vi "CCD photon image_Shaowei.vi"() -> ()   [LabVIEW 2009]
uses:
  <vilib>/Utility/file.llb/Read From Spreadsheet File (DBL).vi
  Instance           5 35Saved   CCD photon image_540_800_CR .vi
  Instance           4 35Saved   CCD photon image_540_800_CR .vi
  Instance           3 35Saved   CCD photon image_540_800_CR .vi
  Instance           8 35Saved   CCD photon image_540_800_CR .vi
  <vilib>/Analysis/Matrix/Numeric/Conversions/Array To Matrix - RA2.vi
  Instance          12 35Saved   CCD photon image_540_800_CR .vi
  Instance          15 35Saved   CCD photon image_540_800_CR .vi
  Instance          18 35Saved   CCD photon image_540_800_CR .vi
  Instance          21 35Saved   CCD photon image_540_800_CR .vi
  Instance          25 35Saved   CCD photon image_540_800_CR .vi
  Instance          24 35Saved   CCD photon image_540_800_CR .vi
  <vilib>/Analysis/Matrix/NI_Matrix.lvlib
panel:
  in  "?":bool
  in  "?":path=path "C:/Users/S. W. Li/Desktop/0463-730.lvm"
  in  "?":path=path "D:/Untitled.txt"
  in  "?":path
  in  "stop 2":bool
  in  "#6":bool
  in  "#5":bool
  in  "?":bool
  in  "stop":bool
  in  "?":ext=1340.0
  in  "to":dbl=950.0
  in  "From":dbl=550.0
  out "Intensity Graph 6":dbl[][](graph)
  out "Col":dbl
  out "to":dbl
  out "Matrix 6":string
  in  "lstart (nm)":dbl
  in  "lend (nm)":dbl
  out "eV":dbl
  out "eV":dbl
  out "Intensity Graph 5":dbl[][](graph)
  out "Col":dbl
  out "to":dbl
  out "Matrix 5":string
  in  "lstart (nm)":dbl
  in  "lend (nm)":dbl
  out "eV":dbl
  out "eV":dbl
  in  "?":bool
  out "MAX":dbl
  out "MIN":dbl
  out "X":sgl
  out "Y":sgl
  out "to":dbl
  out "Col":dbl
  out "eV":dbl
  out "eV":dbl
  in  "lend (nm)":dbl
  in  "lstart (nm)":dbl
  out "eV":dbl
  out "eV":dbl
  in  "lend (nm)":dbl
  in  "lstart (nm)":dbl
  out "to":dbl
  out "Col":dbl
  out "to":dbl
  out "Col":dbl
  out "eV":dbl
  out "eV":dbl
  in  "lend (nm)":dbl
  in  "lstart (nm)":dbl
  in  "?":dbl=32.0
  out "eV":dbl
  out "eV":dbl
  in  "lend (nm)":dbl
  in  "lstart (nm)":dbl
  out "to":dbl
  out "Col":dbl
  in  "#3":bool
  in  "#4":bool
  in  "#2":bool
  out "Intensity Graph 4":dbl[][](graph)
  out "Matrix 4":string
  out "Intensity Graph 3":dbl[][](graph)
  out "Matrix 3":string
  out "Matrix 2":string
  out "Intensity Graph 2":dbl[][](graph)
  out "Matrix 1":string
  out "Intensity Graph":dbl[][](graph)
  # "Input File"
  # "2 Files"
  # "1 File"
  # "1st"
  # "2nd"
  # "Spectra Range"
  # "nm"
  # "nm"
  # "# of Pixel"
  # "Image Size"
  # "Bit"
  # "Active Matrix"
  # "ON"
  # "OFF"
  # "Cosmic Ray Removal"
  # "NO"
  # "YES"
  # "Value"
  # "Position"
  # "Save File"
  # "NO"
  # "YES"
  # "File Name"
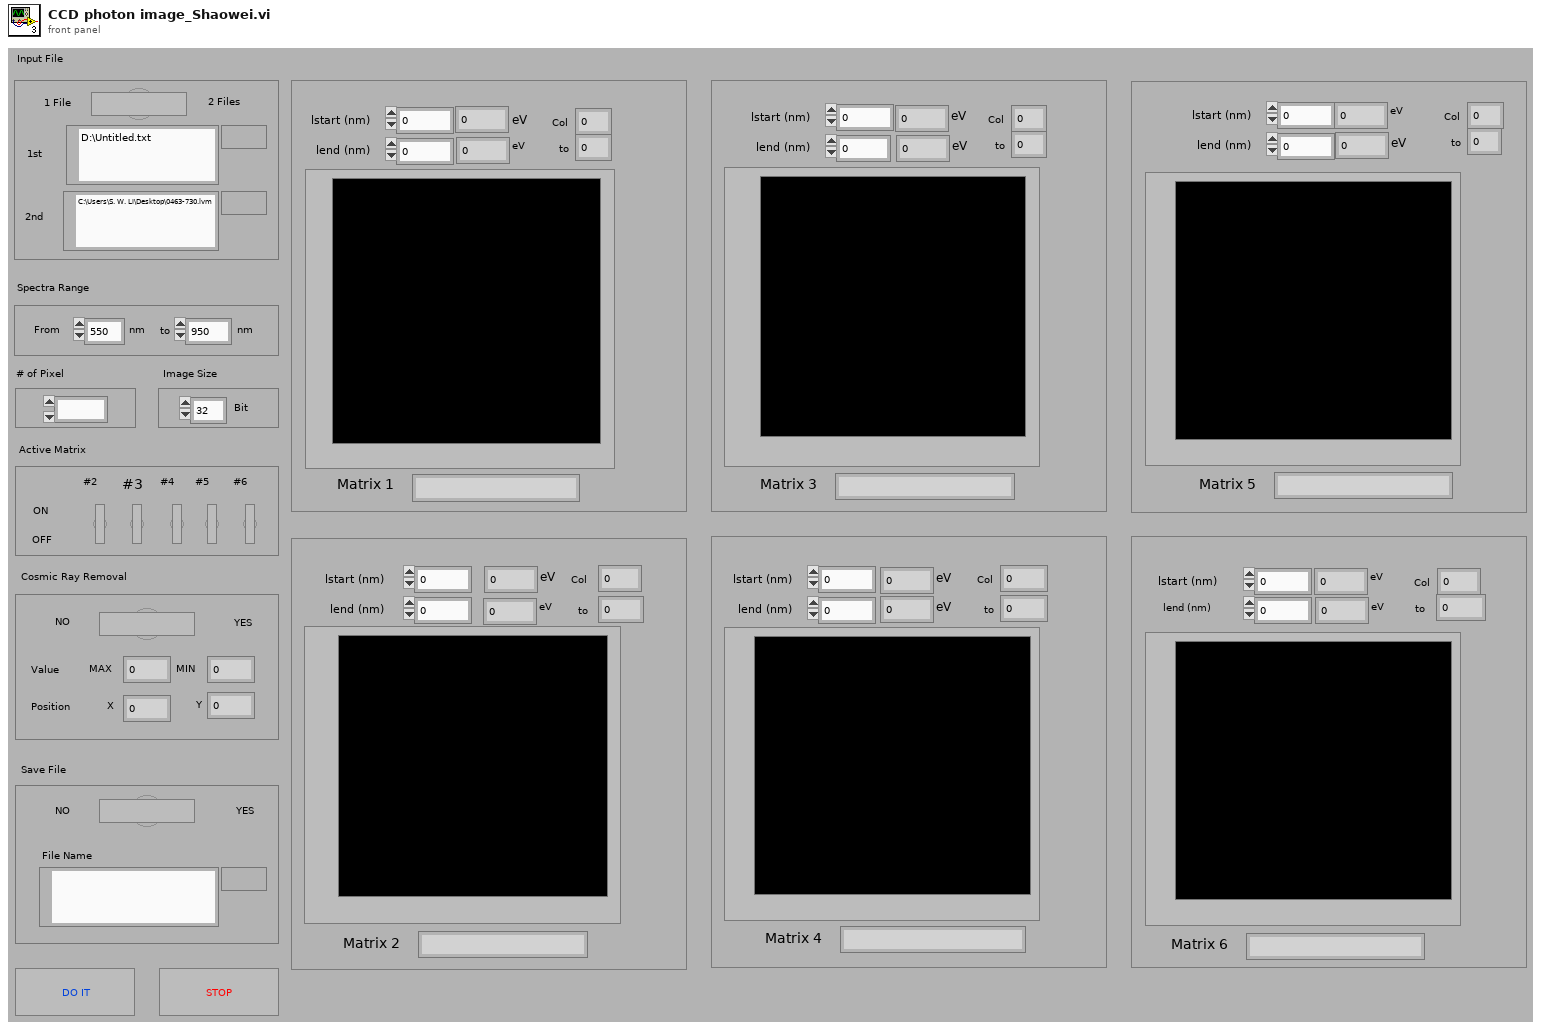
[diagram p1: front panel]
types:
  T1 = typedef "NI_Matrix.lvlib/RealMatrix.ctl" = dbl[][]
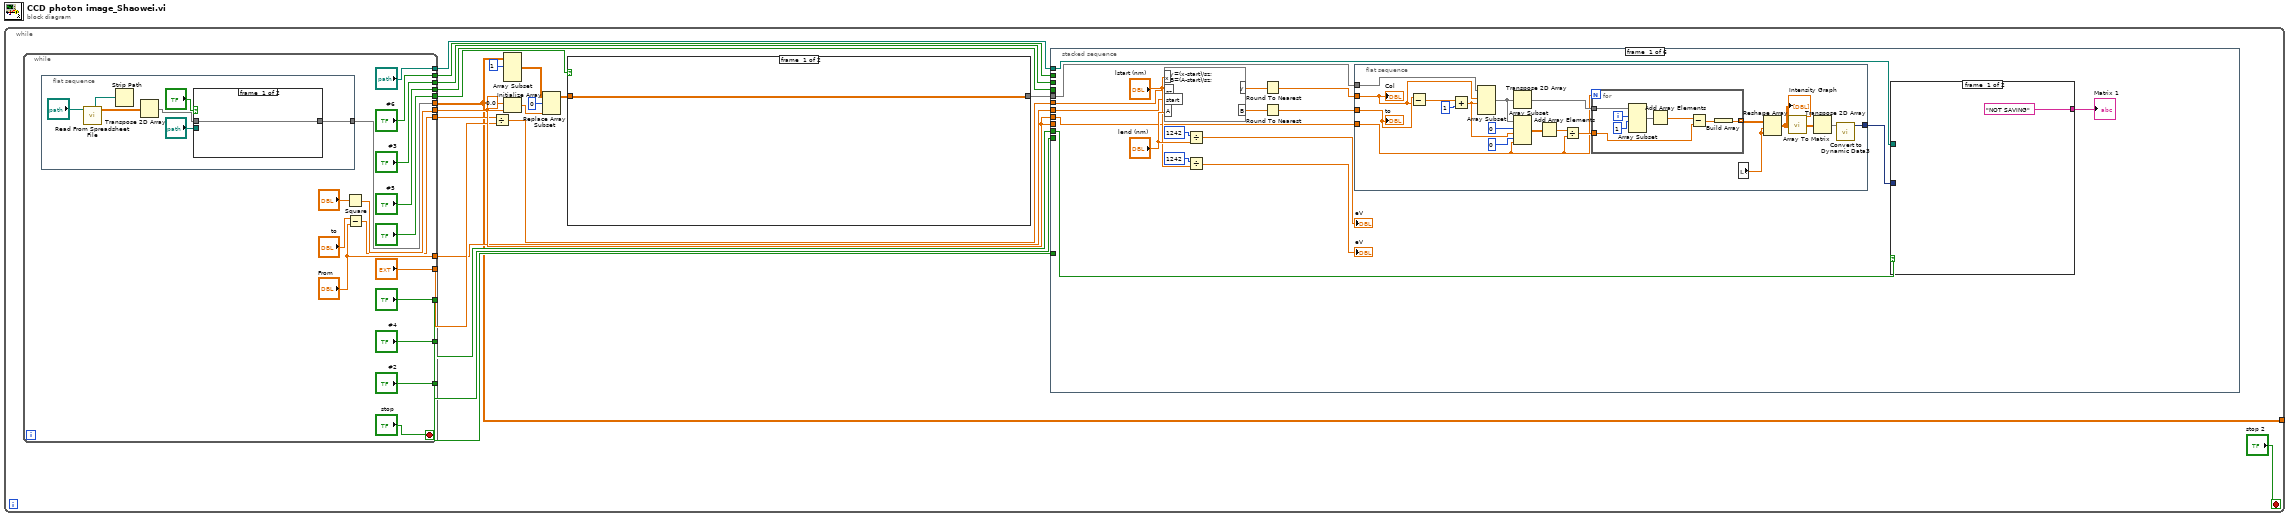
[diagram p0: block diagram]
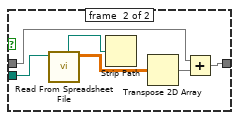
[diagram p2: hidden frame]
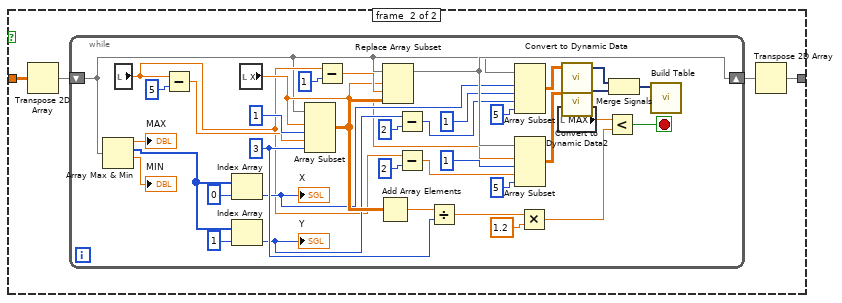
[diagram p3: hidden frame]
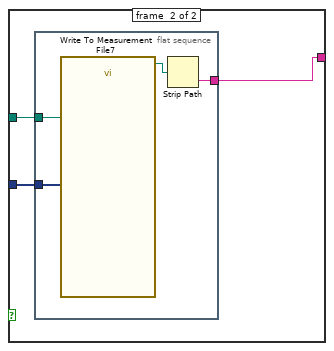
[diagram p4: hidden frame]
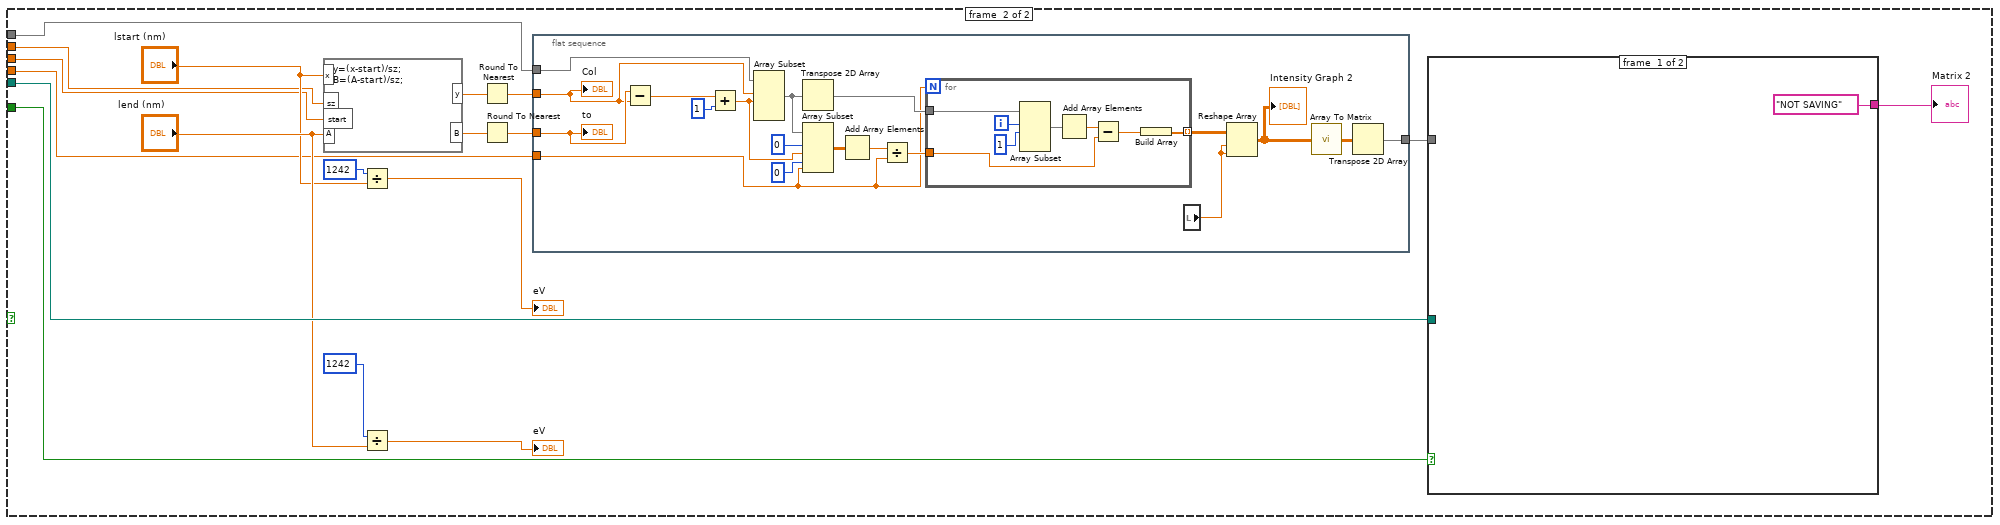
[diagram p6: hidden frame]
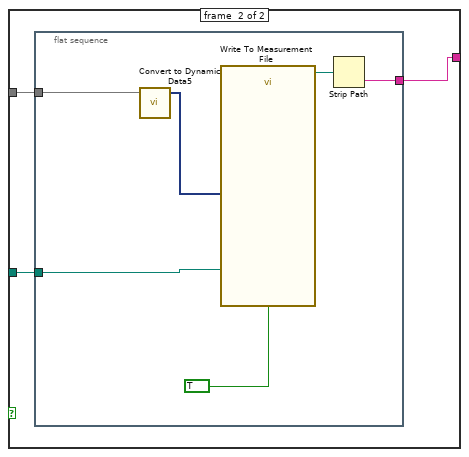
[diagram p7: hidden frame]
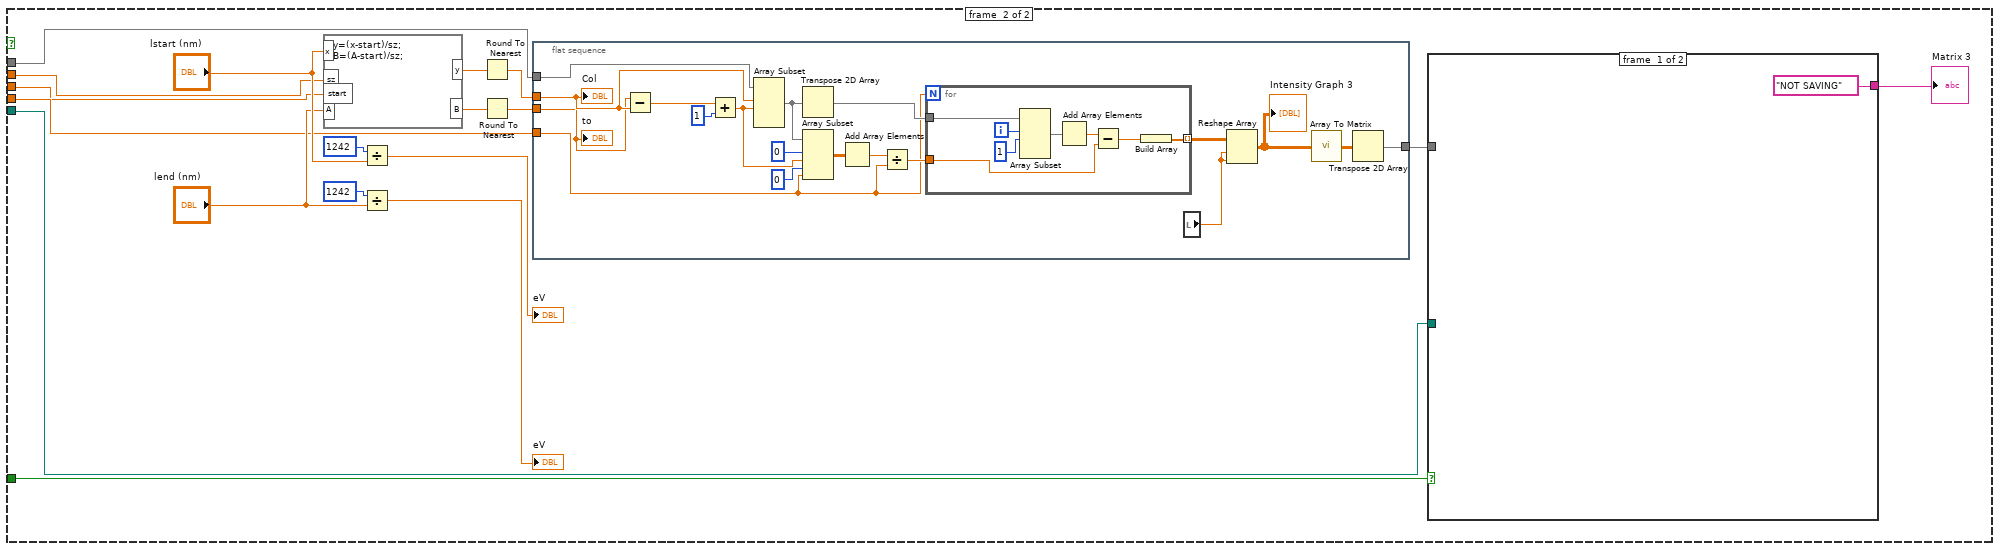
[diagram p9: hidden frame]
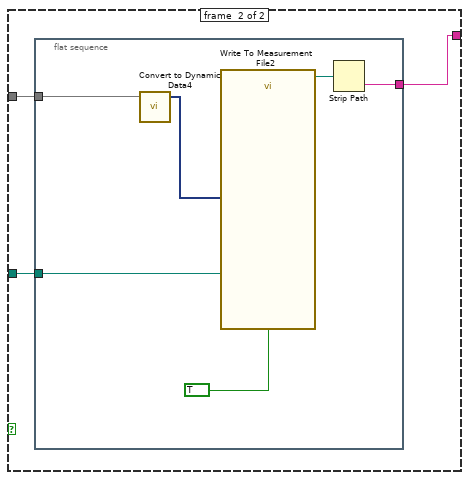
[diagram p10: hidden frame]
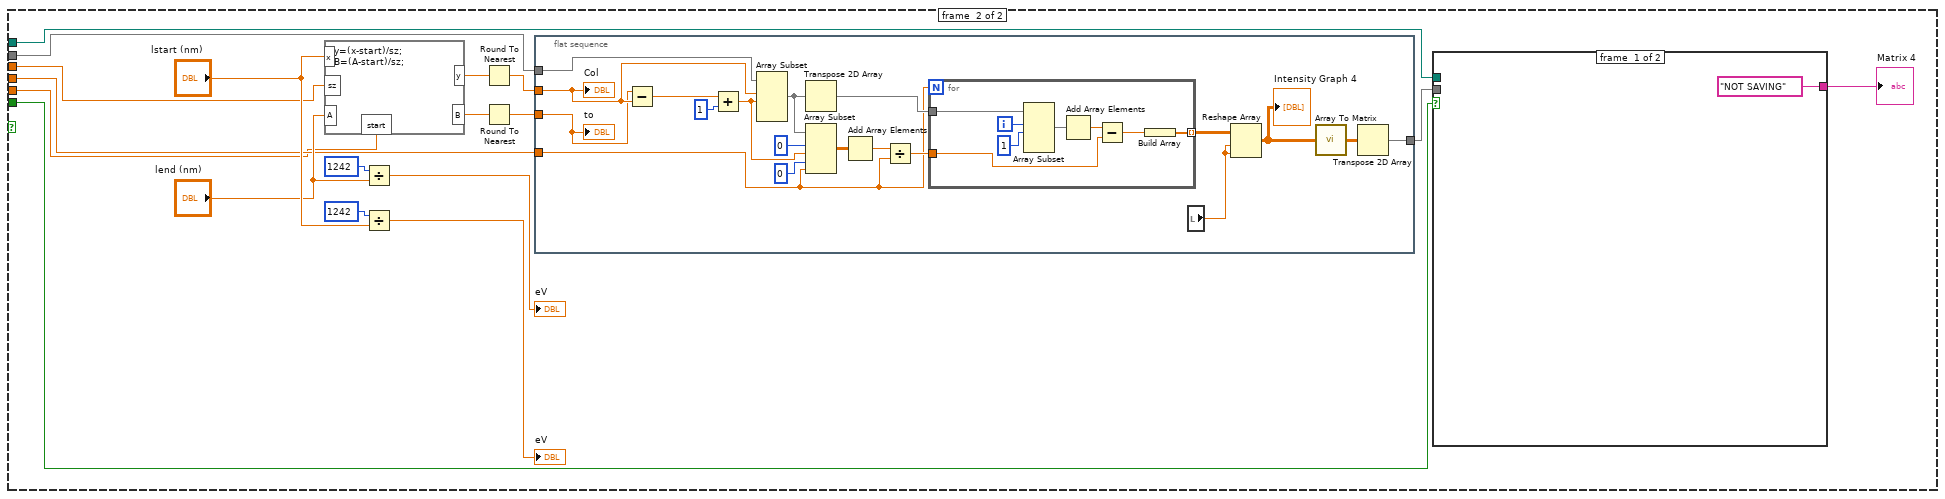
[diagram p12: hidden frame]
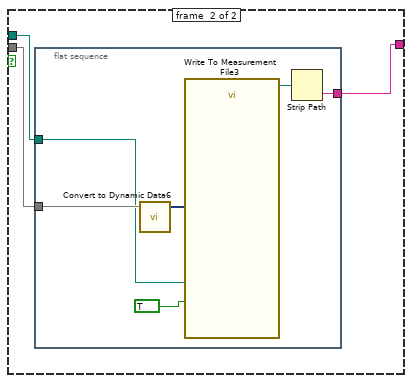
[diagram p13: hidden frame]
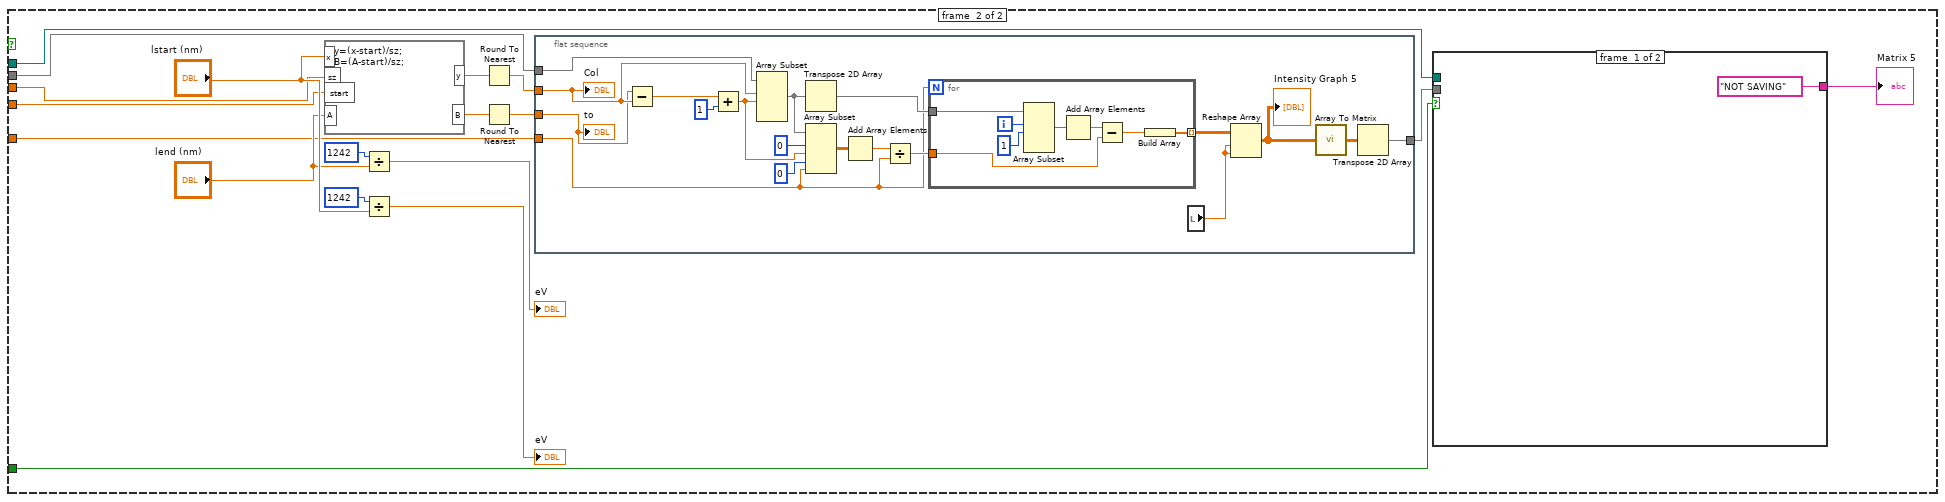
[diagram p15: hidden frame]
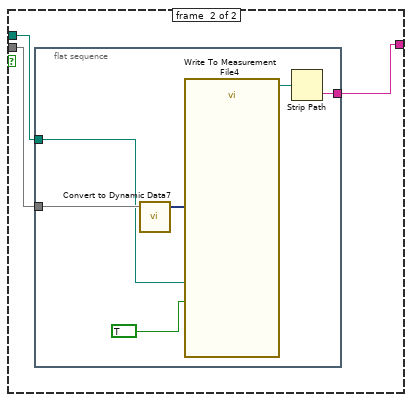
[diagram p16: hidden frame]
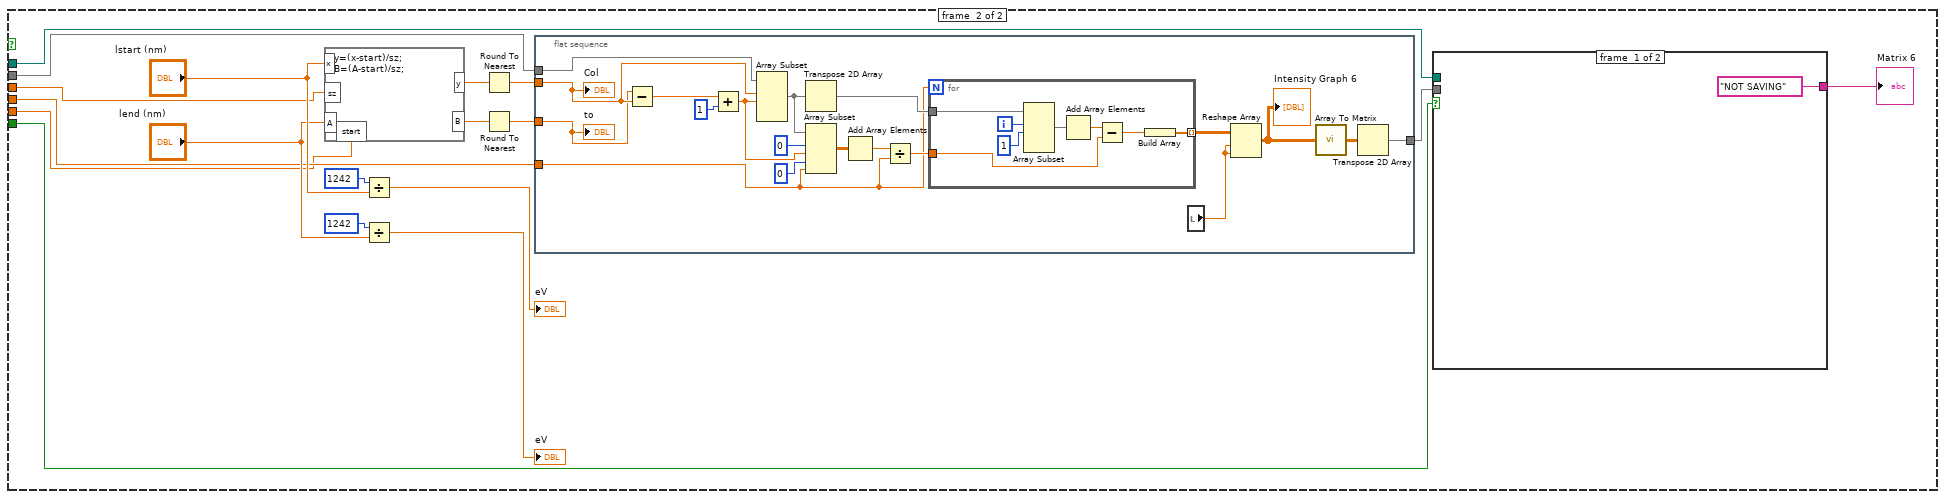
[diagram p18: hidden frame]
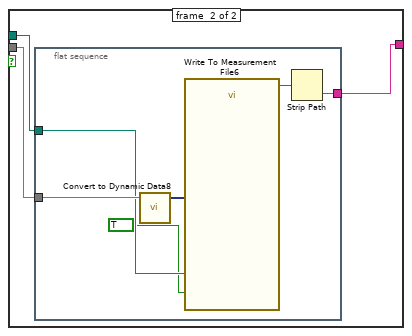
[diagram p19: hidden frame]
diagram:
  n1 = while {
    tunnel: [w2] -> _
    stop <- "stop 2" stop-if-true
    n2 = while {
      tunnel: ["?"] -> w1
      tunnel: ["#4"] -> w22
      tunnel: ["#3"] -> w21
      tunnel: ["#2"] -> w20
      tunnel: [w34] -> w14
      tunnel: ["?"] -> w11
      tunnel: ["?"] -> w10
      tunnel: [w30] -> w9
      tunnel: ["From"] -> w3
      tunnel: ["?"] -> w7
      tunnel: ["#5"] -> w6
      tunnel: ["#6"] -> w5
      tunnel: [w23] -> w2
      stop <- "stop" stop-if-true
      n3 = flat-sequence {
        tunnel: [w42] -> w23
        frame #0 {
          n4 = call-poly <vilib>:"Read From Spreadsheet File.vi"("file path (dialog if empty)"="?") -> ("all rows"=w45:dbl[][], "new file path (Not A Path if cancelled)"=w44:path)  [unwired: 6 in, 3 out]
          n5 = Strip Path(path=w44) -> ()  [unwired: 2 out]
          n6 = Transpose 2D Array(2D array=w45) -> (transposed array=w43:dbl[][])
          n7 = case shown="True" "?" {
            tunnel: w43 -> [w46 w51]
            tunnel: [w46 w50] -> w42
            tunnel: "?" -> [_ w47]
            frame #0 {
            }
            frame #1 {
              n8 = call-poly <vilib>:"Read From Spreadsheet File.vi"("file path (dialog if empty)"=w47) -> ("all rows"=w49:dbl[][], "new file path (Not A Path if cancelled)"=w52:path)  [unwired: 6 in, 3 out]
              n9 = Strip Path(path=w52) -> ()  [unwired: 2 out]
              n10 = Transpose 2D Array(2D array=w49) -> (transposed array=w48:dbl[][])
              n11 = Add(x=w51, y=w48) -> (x+y=w50:dbl[][])
            }
          }
        }
      }
      n12 = Square(x="?") -> (x^2=w34:dbl)
      n13 = Subtract(x="to", y="From") -> (x-y=w30:dbl)
    }
    n14 = Divide(x=w9, y=w10) -> (x/y=w8:ext)
    n15 = Array Subset(array=w2, index (row)=1) -> (w16:dbl[][])  [unwired: 3 in]
    n16 = Initialize Array(0.0 ("element"), w14) -> (w18:dbl[])
    n17 = Replace Array Subset(array=w16, new element=w18, index (row)=0) -> (w13:dbl[][])  [unwired: 1 in]
    n18 = case shown="True" w11 {
      tunnel: w13 -> [w53 w57]
      tunnel: [w53 w55] -> w12
      frame #0 {
      }
      frame #1 {
        n19 = Transpose 2D Array(2D array=w57) -> (transposed array=w56:dbl[][])
        n20 = while {
          shift-right: [w94] -> w54
          shift-left: w56 -> [w58]
          stop <- w73 stop-if-true
          w71 = 3
          n21 = Array Max & Min(array=w58) -> (max value=→"MAX":dbl, max index (indices)=w92:i32[], min value=→"MIN":dbl)  [unwired: 1 out]
          n22 = local read "Y"() -> (w60:sgl)
          n23 = Subtract(x=w60, y=5) -> (x-y=w88:sgl)
          n24 = Index Array(array=w92, index=0) -> (element=w65:i32)
          "X" <- w65
          n25 = Index Array(array=w92, index=1) -> (element=w64:i32)
          "Y" <- w64
          n26 = local read "X"() -> (w61:sgl)
          n27 = Array Subset(array=w58, index (row)=w61, length (row)=1, index (col)=w88, length (col)=w71) -> (w70:dbl[][])
          n28 = Subtract(x=w60, y=1) -> (x-y=w87:sgl)
          n29 = Add Array Elements(numeric array=w70) -> (sum=w72:dbl)
          n30 = Replace Array Subset(array=w58, new element=w70, index (row)=w61, index (col)=w87) -> (w94:dbl[][])
          n31 = Subtract(x=w64, y=2) -> (x-y=w78:i32)
          n32 = Subtract(x=w60, y=2) -> (x-y=w83:sgl)
          n33 = Divide(x=w72, y=w71) -> (x/y=w69:dbl)
          n34 = Array Subset(array=w58, index (row)=w65, length (row)=1, index (col)=w78, length (col)=5) -> (w76:dbl[][])
          n35 = Array Subset(array=w94, index (row)=w61, length (row)=1, index (col)=w83, length (col)=5) -> (w81:dbl[][])
          n36 = Multiply(x=w69, y=1.2) -> (x*y=w74:dbl)
          n37 = local read "MAX"() -> (w59:dbl)
          n38 = call "Convert to Dynamic Data"("2D Array"=w76) -> ("Dynamic Data Type"=w68:dynamicdata)  [unwired: 3 in]
          n39 = call "Convert to Dynamic Data2"("2D Array"=w81) -> ("Dynamic Data Type"=w66:dynamicdata)  [unwired: 3 in]
          n40 = Less?(x=w59, y=w74) -> (x < y?=w73:bool)
          n41 = Merge Signals(w68, w66) -> (w67:dynamicdata)
          n42 = call "Build Table"("Signals"=w67) -> ()  [unwired: 9 in, 2 out]
        }
        n43 = Transpose 2D Array(2D array=w54) -> (transposed array=w55:dbl[][])
      }
    }
    n44 = stacked-sequence {
      tunnel: w1 -> [w112 w155 w217 w279 w341 w403]
      tunnel: w22 -> [_ _ _ w278 _ _]
      tunnel: w21 -> [_ _ w216 _ _ _]
      tunnel: w20 -> [_ w154 _ _ _ _]
      tunnel: w14 -> [w101 w153 w215 _ _ _]
      tunnel: w12 -> [w100 w152 w214 w276 w339 w401]
      tunnel: w14 -> [_ _ _ w277 w340 w402]
      tunnel: w8 -> [w98 w151 w213 w274 w338 w400]
      tunnel: w3 -> [w97 w150 w212 w275 w337 w399]
      tunnel: w7 -> [w96 w149 w211 w273 w336 w398]
      tunnel: w6 -> [_ _ _ _ w335 _]
      tunnel: w5 -> [_ _ _ _ _ w397]
      frame #0 {
        n45 = formula code="y=(x-start)/sz;\nB=(A-start)/sz;"("x"="lstart (nm)", "A"="lend (nm)", "sz"=w98, "start"=w97) -> ("y"=w105:dbl, "B"=w104:dbl)
        n46 = Divide(x=1242, y="lend (nm)") -> (x/y=→"eV":dbl)
        n47 = Divide(x=1242, y="lstart (nm)") -> (x/y=→"eV":dbl)
        n48 = Round To Nearest(number=w105) -> (nearest integer value=w103:dbl)
        n49 = Round To Nearest(number=w104) -> (nearest integer value=w102:dbl)
        n50 = flat-sequence {
          tunnel: [w140] -> w99
          tunnel: w102 -> [w133]
          tunnel: w103 -> [w132]
          tunnel: w101 -> [w121]
          tunnel: w100 -> [w125]
          frame #0 {
            n51 = Subtract(x=w133, y=w132) -> (x-y=w128:dbl)
            n52 = Add(x=w128, y=1) -> (x+y=w126:dbl)
            n53 = Array Subset(array=w125, index (row)=w132, length (row)=w126) -> (w124:dbl[][])  [unwired: 2 in]
            n54 = Transpose 2D Array(2D array=w124) -> (transposed array=w135:dbl[][])
            n55 = Array Subset(array=w124, index (row)=0, length (row)=w126, index (col)=0, length (col)=w121) -> (w123:dbl[][])
            n56 = Add Array Elements(numeric array=w123) -> (sum=w129:dbl)
            n57 = Divide(x=w129, y=w121) -> (x/y=w127:dbl)
            n58 = for {
              N: w121 -> [_]
              tunnel: w135 -> [w142]
              tunnel: [w144] -> w134 mode=indexing
              tunnel: w127 -> [w143]
              i -> [w148]
              n59 = Array Subset(array=w142, index (row)=w148, length (row)=1) -> (w141:dbl[][])  [unwired: 2 in]
              n60 = Add Array Elements(numeric array=w141) -> (sum=w146:dbl)
              n61 = Subtract(x=w146, y=w143) -> (x-y=w145:dbl)
              n62 = Build Array(w145) -> (w144:dbl[])
            }
            n63 = local read item#17() -> (w122:dbl)
            n64 = Reshape Array(w134, w122, w122) -> (w136:dbl[][])
            "Intensity Graph" <- w136
            n65 = call-poly <vilib>:"Array To Matrix.vi"("Real 2D Array"=w136) -> ("Real Matrix"=w139:T1)
            n66 = Transpose 2D Array(2D array=w139) -> (transposed array=w138:T1)
            n67 = call "Convert to Dynamic Data3"("2D Array"=w138) -> ("Dynamic Data Type"=w140:dynamicdata)  [unwired: 3 in]
            "Col" <- w132
            "to" <- w133
          }
        }
        n68 = case shown="False" w96 {
          tunnel: w112 -> [_ w116]
          tunnel: w99 -> [_ w115]
          tunnel: ["NOT SAVING" w114] -> w95
          frame #0 {
          }
          frame #1 {
            n69 = flat-sequence {
              tunnel: w116 -> [w118]
              tunnel: w115 -> [w119]
              tunnel: [w117] -> w114
              frame #0 {
                n70 = call "Write To Measurement File7"("Signals"=w119, "Filename"=w118) -> ("Filename Out"=w120:path)  [unwired: 15 in, 2 out]
                n71 = Strip Path(path=w120) -> (name=w117:string)  [unwired: 1 out]
              }
            }
          }
        }
        "Matrix 1" <- w95
      }
      frame #1 {
        n72 = case shown="True" w154 {
          tunnel: w155 -> [_ w172]
          tunnel: w153 -> [_ w161]
          tunnel: w152 -> [_ w160]
          tunnel: w151 -> [_ w159]
          tunnel: w150 -> [_ w158]
          tunnel: w149 -> [_ w157]
          frame #0 {
          }
          frame #1 {
            n73 = formula code="y=(x-start)/sz;\nB=(A-start)/sz;"("x"="lstart (nm)", "A"="lend (nm)", "sz"=w159, "start"=w158) -> ("y"=w165:dbl, "B"=w164:dbl)
            n74 = Divide(x=1242, y="lstart (nm)") -> (x/y=→"eV":dbl)
            n75 = Divide(x=1242, y="lend (nm)") -> (x/y=→"eV":dbl)
            n76 = Round To Nearest(number=w165) -> (nearest integer value=w163:dbl)
            n77 = Round To Nearest(number=w164) -> (nearest integer value=w162:dbl)
            n78 = flat-sequence {
              tunnel: w163 -> [w189]
              tunnel: w162 -> [w190]
              tunnel: [w197] -> w173
              tunnel: w161 -> [w185]
              tunnel: w160 -> [w184]
              frame #0 {
                n79 = Subtract(x=w190, y=w189) -> (x-y=w198:dbl)
                n80 = Add(x=w198, y=1) -> (x+y=w192:dbl)
                n81 = Array Subset(array=w184, index (row)=w189, length (row)=w192) -> (w188:dbl[][])  [unwired: 2 in]
                n82 = Transpose 2D Array(2D array=w188) -> (transposed array=w201:dbl[][])
                n83 = Array Subset(array=w188, index (row)=0, length (row)=w192, index (col)=0, length (col)=w185) -> (w186:dbl[][])
                n84 = Add Array Elements(numeric array=w186) -> (sum=w195:dbl)
                n85 = Divide(x=w195, y=w185) -> (x/y=w191:dbl)
                n86 = for {
                  N: w185 -> [_]
                  tunnel: w201 -> [w210]
                  tunnel: [w203] -> w202 mode=indexing
                  tunnel: w191 -> [w205]
                  i -> [w209]
                  n87 = Array Subset(array=w210, index (row)=w209, length (row)=1) -> (w208:dbl[][])  [unwired: 2 in]
                  n88 = Add Array Elements(numeric array=w208) -> (sum=w206:dbl)
                  n89 = Subtract(x=w206, y=w205) -> (x-y=w204:dbl)
                  n90 = Build Array(w204) -> (w203:dbl[])
                }
                n91 = local read item#17() -> (w187:dbl)
                n92 = Reshape Array(w202, w187, w187) -> (w200:dbl[][])
                "Intensity Graph 2" <- w200
                n93 = call-poly <vilib>:"Array To Matrix.vi"("Real 2D Array"=w200) -> ("Real Matrix"=w196:T1)
                n94 = Transpose 2D Array(2D array=w196) -> (transposed array=w197:T1)
                "Col" <- w189
                "to" <- w190
              }
            }
            n95 = case shown="True" w157 {
              tunnel: w173 -> [_ w177]
              tunnel: w172 -> [_ w176]
              tunnel: ["NOT SAVING" w175] -> w156
              frame #0 {
              }
              frame #1 {
                n96 = flat-sequence {
                  tunnel: w177 -> [w183]
                  tunnel: w176 -> [w180]
                  tunnel: [w179] -> w175
                  frame #0 {
                    n97 = call "Convert to Dynamic Data5"("2D Array"=w183) -> ("Dynamic Data Type"=w181:dynamicdata)  [unwired: 3 in]
                    n98 = call "Write To Measurement File"("Signals"=w181, "Reset"=TRUE, "Filename"=w180) -> ("Filename Out"=w182:path)  [unwired: 14 in, 2 out]
                    n99 = Strip Path(path=w182) -> (name=w179:string)  [unwired: 1 out]
                  }
                }
              }
            }
            "Matrix 2" <- w156
          }
        }
      }
      frame #2 {
        n100 = case shown="True" w216 {
          tunnel: w217 -> [_ w234]
          tunnel: w215 -> [_ w223]
          tunnel: w214 -> [_ w222]
          tunnel: w213 -> [_ w221]
          tunnel: w212 -> [_ w220]
          tunnel: w211 -> [_ w219]
          frame #0 {
          }
          frame #1 {
            n101 = formula code="y=(x-start)/sz;\nB=(A-start)/sz;"("x"="lstart (nm)", "A"="lend (nm)", "sz"=w221, "start"=w220) -> ("y"=w231:dbl, "B"=w230:dbl)
            n102 = Divide(x=1242, y="lstart (nm)") -> (x/y=→"eV":dbl)
            n103 = Divide(x=1242, y="lend (nm)") -> (x/y=→"eV":dbl)
            n104 = Round To Nearest(number=w231) -> (nearest integer value=w229:dbl)
            n105 = Round To Nearest(number=w230) -> (nearest integer value=w228:dbl)
            n106 = flat-sequence {
              tunnel: w228 -> [w251]
              tunnel: w229 -> [w252]
              tunnel: [w259] -> w235
              tunnel: w223 -> [w247]
              tunnel: w222 -> [w246]
              frame #0 {
                n107 = Subtract(x=w251, y=w252) -> (x-y=w260:dbl)
                n108 = Add(x=w260, y=1) -> (x+y=w254:dbl)
                n109 = Array Subset(array=w246, index (row)=w252, length (row)=w254) -> (w248:dbl[][])  [unwired: 2 in]
                n110 = Transpose 2D Array(2D array=w248) -> (transposed array=w263:dbl[][])
                n111 = Array Subset(array=w248, index (row)=0, length (row)=w254, index (col)=0, length (col)=w247) -> (w249:dbl[][])
                n112 = Add Array Elements(numeric array=w249) -> (sum=w255:dbl)
                n113 = Divide(x=w255, y=w247) -> (x/y=w253:dbl)
                n114 = for {
                  N: w247 -> [_]
                  tunnel: w263 -> [w272]
                  tunnel: [w266] -> w264 mode=indexing
                  tunnel: w253 -> [w265]
                  i -> [w271]
                  n115 = Array Subset(array=w272, index (row)=w271, length (row)=1) -> (w270:dbl[][])  [unwired: 2 in]
                  n116 = Add Array Elements(numeric array=w270) -> (sum=w268:dbl)
                  n117 = Subtract(x=w268, y=w265) -> (x-y=w267:dbl)
                  n118 = Build Array(w267) -> (w266:dbl[])
                }
                n119 = local read item#17() -> (w250:dbl)
                n120 = Reshape Array(w264, w250, w250) -> (w262:dbl[][])
                "Intensity Graph 3" <- w262
                n121 = call-poly <vilib>:"Array To Matrix.vi"("Real 2D Array"=w262) -> ("Real Matrix"=w258:T1)
                n122 = Transpose 2D Array(2D array=w258) -> (transposed array=w259:T1)
                "Col" <- w252
                "to" <- w251
              }
            }
            n123 = case shown="True" w219 {
              tunnel: w235 -> [_ w239]
              tunnel: w234 -> [_ w238]
              tunnel: ["NOT SAVING" w237] -> w218
              frame #0 {
              }
              frame #1 {
                n124 = flat-sequence {
                  tunnel: w239 -> [w245]
                  tunnel: w238 -> [w242]
                  tunnel: [w241] -> w237
                  frame #0 {
                    n125 = call "Convert to Dynamic Data4"("2D Array"=w245) -> ("Dynamic Data Type"=w243:dynamicdata)  [unwired: 3 in]
                    n126 = call "Write To Measurement File2"("Signals"=w243, "Reset"=TRUE, "Filename"=w242) -> ("Filename Out"=w244:path)  [unwired: 14 in, 2 out]
                    n127 = Strip Path(path=w244) -> (name=w241:string)  [unwired: 1 out]
                  }
                }
              }
            }
            "Matrix 3" <- w218
          }
        }
      }
      frame #3 {
        n128 = case shown="True" w278 {
          tunnel: w279 -> [_ w296]
          tunnel: w277 -> [_ w285]
          tunnel: w276 -> [_ w284]
          tunnel: w275 -> [_ w283]
          tunnel: w274 -> [_ w282]
          tunnel: w273 -> [_ w281]
          frame #0 {
          }
          frame #1 {
            n129 = formula code="y=(x-start)/sz;\nB=(A-start)/sz;"("x"="lstart (nm)", "A"="lend (nm)", "sz"=w282, "start"=w283) -> ("y"=w293:dbl, "B"=w292:dbl)
            n130 = Divide(x=1242, y="lend (nm)") -> (x/y=→"eV":dbl)
            n131 = Divide(x=1242, y="lstart (nm)") -> (x/y=→"eV":dbl)
            n132 = Round To Nearest(number=w293) -> (nearest integer value=w287:dbl)
            n133 = Round To Nearest(number=w292) -> (nearest integer value=w286:dbl)
            n134 = flat-sequence {
              tunnel: w287 -> [w315]
              tunnel: w286 -> [w314]
              tunnel: [w322] -> w297
              tunnel: w285 -> [w308]
              tunnel: w284 -> [w309]
              frame #0 {
                n135 = Subtract(x=w314, y=w315) -> (x-y=w323:dbl)
                n136 = Add(x=w323, y=1) -> (x+y=w316:dbl)
                n137 = Array Subset(array=w309, index (row)=w315, length (row)=w316) -> (w313:dbl[][])  [unwired: 2 in]
                n138 = Transpose 2D Array(2D array=w313) -> (transposed array=w312:dbl[][])
                n139 = Array Subset(array=w313, index (row)=0, length (row)=w316, index (col)=0, length (col)=w308) -> (w310:dbl[][])
                n140 = Add Array Elements(numeric array=w310) -> (sum=w318:dbl)
                n141 = Divide(x=w318, y=w308) -> (x/y=w317:dbl)
                n142 = for {
                  N: w308 -> [_]
                  tunnel: w312 -> [w334]
                  tunnel: [w328] -> w326 mode=indexing
                  tunnel: w317 -> [w327]
                  i -> [w333]
                  n143 = Array Subset(array=w334, index (row)=w333, length (row)=1) -> (w332:dbl[][])  [unwired: 2 in]
                  n144 = Add Array Elements(numeric array=w332) -> (sum=w330:dbl)
                  n145 = Subtract(x=w330, y=w327) -> (x-y=w329:dbl)
                  n146 = Build Array(w329) -> (w328:dbl[])
                }
                n147 = local read item#17() -> (w311:dbl)
                n148 = Reshape Array(w326, w311, w311) -> (w325:dbl[][])
                "Intensity Graph 4" <- w325
                n149 = call-poly <vilib>:"Array To Matrix.vi"("Real 2D Array"=w325) -> ("Real Matrix"=w321:T1)
                n150 = Transpose 2D Array(2D array=w321) -> (transposed array=w322:T1)
                "Col" <- w315
                "to" <- w314
              }
            }
            n151 = case shown="True" w281 {
              tunnel: w297 -> [_ w301]
              tunnel: w296 -> [_ w300]
              tunnel: ["NOT SAVING" w299] -> w280
              frame #0 {
              }
              frame #1 {
                n152 = flat-sequence {
                  tunnel: w301 -> [w307]
                  tunnel: w300 -> [w304]
                  tunnel: [w303] -> w299
                  frame #0 {
                    n153 = call "Convert to Dynamic Data6"("2D Array"=w307) -> ("Dynamic Data Type"=w305:dynamicdata)  [unwired: 3 in]
                    n154 = call "Write To Measurement File3"("Signals"=w305, "Reset"=TRUE, "Filename"=w304) -> ("Filename Out"=w306:path)  [unwired: 14 in, 2 out]
                    n155 = Strip Path(path=w306) -> (name=w303:string)  [unwired: 1 out]
                  }
                }
              }
            }
            "Matrix 4" <- w280
          }
        }
      }
      frame #4 {
        n156 = case shown="True" w335 {
          tunnel: w341 -> [_ w358]
          tunnel: w340 -> [_ w347]
          tunnel: w339 -> [_ w346]
          tunnel: w338 -> [_ w345]
          tunnel: w337 -> [_ w344]
          tunnel: w336 -> [_ w343]
          frame #0 {
          }
          frame #1 {
            n157 = formula code="y=(x-start)/sz;\nB=(A-start)/sz;"("x"="lstart (nm)", "A"="lend (nm)", "sz"=w345, "start"=w344) -> ("y"=w355:dbl, "B"=w354:dbl)
            n158 = Divide(x=1242, y="lend (nm)") -> (x/y=→"eV":dbl)
            n159 = Divide(x=1242, y="lstart (nm)") -> (x/y=→"eV":dbl)
            n160 = Round To Nearest(number=w355) -> (nearest integer value=w349:dbl)
            n161 = Round To Nearest(number=w354) -> (nearest integer value=w348:dbl)
            n162 = flat-sequence {
              tunnel: w349 -> [w377]
              tunnel: w348 -> [w376]
              tunnel: [w384] -> w359
              tunnel: w347 -> [w370]
              tunnel: w346 -> [w371]
              frame #0 {
                n163 = Subtract(x=w376, y=w377) -> (x-y=w385:dbl)
                n164 = Add(x=w385, y=1) -> (x+y=w378:dbl)
                n165 = Array Subset(array=w371, index (row)=w377, length (row)=w378) -> (w375:dbl[][])  [unwired: 2 in]
                n166 = Transpose 2D Array(2D array=w375) -> (transposed array=w374:dbl[][])
                n167 = Array Subset(array=w375, index (row)=0, length (row)=w378, index (col)=0, length (col)=w370) -> (w372:dbl[][])
                n168 = Add Array Elements(numeric array=w372) -> (sum=w380:dbl)
                n169 = Divide(x=w380, y=w370) -> (x/y=w379:dbl)
                n170 = for {
                  N: w370 -> [_]
                  tunnel: w374 -> [w396]
                  tunnel: [w390] -> w388 mode=indexing
                  tunnel: w379 -> [w389]
                  i -> [w395]
                  n171 = Array Subset(array=w396, index (row)=w395, length (row)=1) -> (w394:dbl[][])  [unwired: 2 in]
                  n172 = Add Array Elements(numeric array=w394) -> (sum=w392:dbl)
                  n173 = Subtract(x=w392, y=w389) -> (x-y=w391:dbl)
                  n174 = Build Array(w391) -> (w390:dbl[])
                }
                n175 = local read item#17() -> (w373:dbl)
                n176 = Reshape Array(w388, w373, w373) -> (w387:dbl[][])
                "Intensity Graph 5" <- w387
                n177 = call-poly <vilib>:"Array To Matrix.vi"("Real 2D Array"=w387) -> ("Real Matrix"=w383:T1)
                n178 = Transpose 2D Array(2D array=w383) -> (transposed array=w384:T1)
                "Col" <- w377
                "to" <- w376
              }
            }
            n179 = case shown="True" w343 {
              tunnel: w359 -> [_ w363]
              tunnel: w358 -> [_ w362]
              tunnel: ["NOT SAVING" w361] -> w342
              frame #0 {
              }
              frame #1 {
                n180 = flat-sequence {
                  tunnel: w363 -> [w369]
                  tunnel: w362 -> [w366]
                  tunnel: [w365] -> w361
                  frame #0 {
                    n181 = call "Convert to Dynamic Data7"("2D Array"=w369) -> ("Dynamic Data Type"=w367:dynamicdata)  [unwired: 3 in]
                    n182 = call "Write To Measurement File4"("Signals"=w367, "Reset"=TRUE, "Filename"=w366) -> ("Filename Out"=w368:path)  [unwired: 14 in, 2 out]
                    n183 = Strip Path(path=w368) -> (name=w365:string)  [unwired: 1 out]
                  }
                }
              }
            }
            "Matrix 5" <- w342
          }
        }
      }
      frame #5 {
        n184 = case shown="True" w397 {
          tunnel: w403 -> [_ w420]
          tunnel: w402 -> [_ w409]
          tunnel: w401 -> [_ w408]
          tunnel: w400 -> [_ w407]
          tunnel: w399 -> [_ w406]
          tunnel: w398 -> [_ w405]
          frame #0 {
          }
          frame #1 {
            n185 = formula code="y=(x-start)/sz;\nB=(A-start)/sz;"("x"="lstart (nm)", "A"="lend (nm)", "sz"=w407, "start"=w406) -> ("y"=w417:dbl, "B"=w416:dbl)
            n186 = Divide(x=1242, y="lstart (nm)") -> (x/y=→"eV":dbl)
            n187 = Divide(x=1242, y="lend (nm)") -> (x/y=→"eV":dbl)
            n188 = Round To Nearest(number=w417) -> (nearest integer value=w411:dbl)
            n189 = Round To Nearest(number=w416) -> (nearest integer value=w410:dbl)
            n190 = flat-sequence {
              tunnel: w411 -> [w439]
              tunnel: w410 -> [w438]
              tunnel: [w446] -> w421
              tunnel: w409 -> [w432]
              tunnel: w408 -> [w433]
              frame #0 {
                n191 = Subtract(x=w438, y=w439) -> (x-y=w447:dbl)
                n192 = Add(x=w447, y=1) -> (x+y=w440:dbl)
                n193 = Array Subset(array=w433, index (row)=w439, length (row)=w440) -> (w437:dbl[][])  [unwired: 2 in]
                n194 = Transpose 2D Array(2D array=w437) -> (transposed array=w436:dbl[][])
                n195 = Array Subset(array=w437, index (row)=0, length (row)=w440, index (col)=0, length (col)=w432) -> (w434:dbl[][])
                n196 = Add Array Elements(numeric array=w434) -> (sum=w442:dbl)
                n197 = Divide(x=w442, y=w432) -> (x/y=w441:dbl)
                n198 = for {
                  N: w432 -> [_]
                  tunnel: w436 -> [w458]
                  tunnel: [w452] -> w450 mode=indexing
                  tunnel: w441 -> [w451]
                  i -> [w457]
                  n199 = Array Subset(array=w458, index (row)=w457, length (row)=1) -> (w456:dbl[][])  [unwired: 2 in]
                  n200 = Add Array Elements(numeric array=w456) -> (sum=w454:dbl)
                  n201 = Subtract(x=w454, y=w451) -> (x-y=w453:dbl)
                  n202 = Build Array(w453) -> (w452:dbl[])
                }
                n203 = local read item#17() -> (w435:dbl)
                n204 = Reshape Array(w450, w435, w435) -> (w449:dbl[][])
                "Intensity Graph 6" <- w449
                n205 = call-poly <vilib>:"Array To Matrix.vi"("Real 2D Array"=w449) -> ("Real Matrix"=w445:T1)
                n206 = Transpose 2D Array(2D array=w445) -> (transposed array=w446:T1)
                "Col" <- w439
                "to" <- w438
              }
            }
            n207 = case shown="True" w405 {
              tunnel: w421 -> [_ w425]
              tunnel: w420 -> [_ w424]
              tunnel: ["NOT SAVING" w423] -> w404
              frame #0 {
              }
              frame #1 {
                n208 = flat-sequence {
                  tunnel: w425 -> [w431]
                  tunnel: w424 -> [w428]
                  tunnel: [w427] -> w423
                  frame #0 {
                    n209 = call "Convert to Dynamic Data8"("2D Array"=w431) -> ("Dynamic Data Type"=w429:dynamicdata)  [unwired: 3 in]
                    n210 = call "Write To Measurement File6"("Reset"=TRUE, "File Name"=w428, "Signals"=w429) -> ("File Name Out"=w430:path)  [unwired: 6 in, 2 out]
                    n211 = Strip Path(path=w430) -> (name=w427:string)  [unwired: 1 out]
                  }
                }
              }
            }
            "Matrix 6" <- w404
          }
        }
      }
    }
  }
